vi "Global_Variable_Status_Indicator.vi"() -> ()   [LabVIEW 2017]
panel:
  in  "Stop welding":bool
  out "Pre Part contanct in inch":dbl
  out "Absolute distance in inch":dbl
  out "Pre part contanct in mm":dbl
  out "Absolute distance in mm":dbl
  out "Status Indicator":string
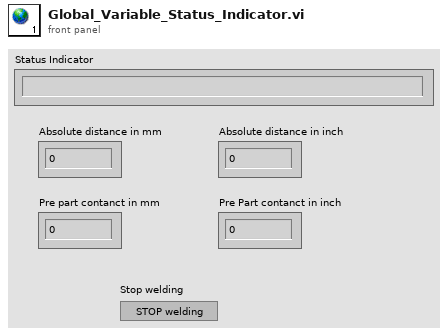
[diagram p1: front panel]
diagram:
